vi "SetMatlabBoundControlCollection.vi"(10 "Bound controls":T1[](array[typedef]), 11 "ExpID":string="ThisISATestColID") -> ()   [LabVIEW 2017]
uses:
  Types/ControlValueChangeEventBindingType.ctl
  Types/MatlabBindingDirectionEnum.ctl
  MatlabGlobals.vi
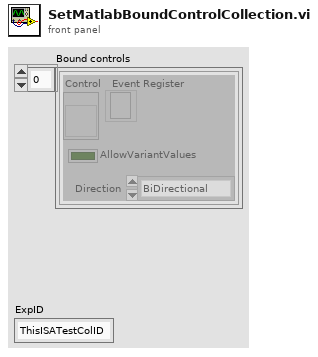
[diagram p1: front panel]
types:
  T1 = typedef "ControlValueChangeEventBindingType.ctl" = cluster{"Control":refnum<vi>, "Event Register":refnum<event-registration>, "AllowVariantValues":bool, "Direction":T2}
  T2 = typedef "MatlabBindingDirectionEnum.ctl" = enum16{"BiDirectional", "FromMatlab", "ToMatlab"}
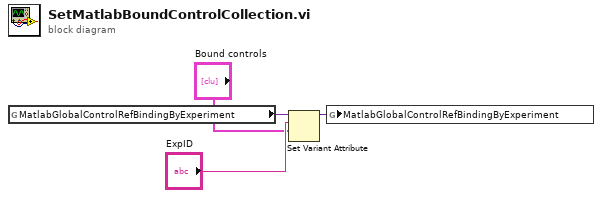
[diagram p0: block diagram]
diagram:
  n1 = global read "MatlabGlobals.vi" "MatlabGlobalControlRefBindingByExperiment"() -> (w2:variant)
  n2 = Set Variant Attribute(Variant=w2, name="ExpID", value="Bound controls") -> (Variant out=w4:variant)  [unwired: 1 in, 2 out]
  n3 = global write "MatlabGlobals.vi" "MatlabGlobalControlRefBindingByExperiment"(w4) -> ()
